vi "Write Sensor Servo Offset.vi"(7 "save to file (F)":bool, 8 "error in (no error)":errorcluster, 10 "ccw offset angle (rad)":dbl, 11 "starter kit host in":refnum<class "NI_Robotics_Starter Kit Host.lvclass">) -> (0 "error out":errorcluster, 3 "starter kit host out":refnum<class "NI_Robotics_Starter Kit Host.lvclass">)   [LabVIEW 2017, in "NI_Robotics_Starter Kit Host.lvclass"]
doc: "<B>Owning Palette:</B> Starter Kit 1.0 VIs, Starter Kit 2.0 VIs\n\nDefines the amount by which the zero, or straight-forward, position of the distance sensor differs from the zero position of the sensor servo on which the sensor is mounted. You can use this VI to save the offset value to a file so the value is associated with the same robot in the future."
uses:
  <vilib>/robotics/Starter Kit/Host Interface/NI_Robotics_Starter Kit Host.lvclass
  <vilib>/robotics/Starter Kit/Host Interface/NI_Robotics_Starter Kit Host.lvclass/NI_Robotics_Starter Kit Host.ctl
  <vilib>/robotics/Starter Kit/Servo Motor/NI_Robotics_Starter Kit Servo Motor.lvclass
  <vilib>/robotics/Utilities/NI_Robotics Utilities.lvlib
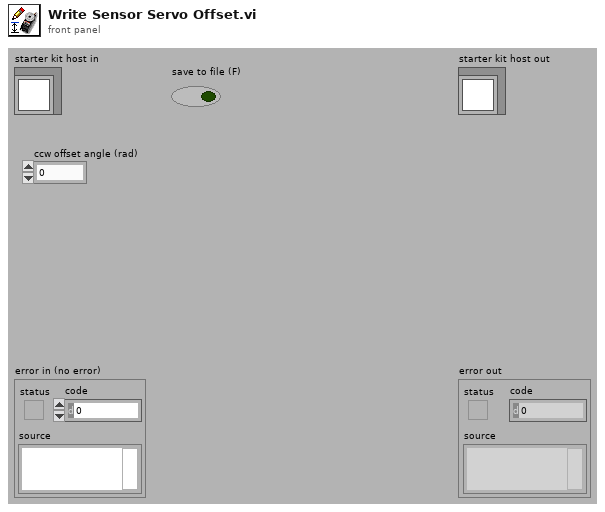
[diagram p1: front panel]
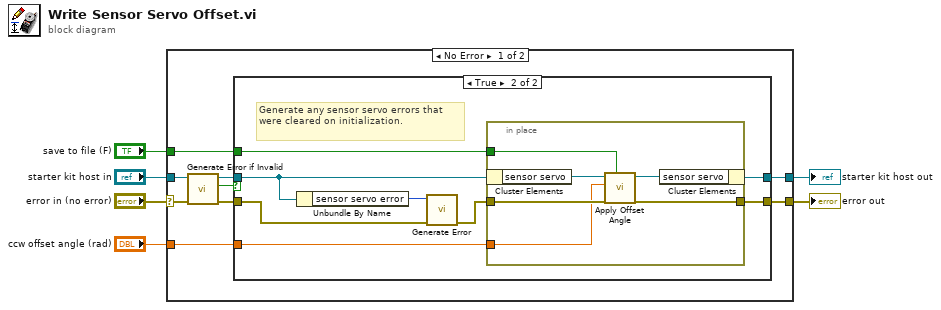
[diagram p0: block diagram]
diagram:
  n1 = case shown="No Error" "error in (no error)" {
    selector: "error in (no error)" -> [w9 w33]
    tunnel: [w14 w33] -> w5
    tunnel: [w15 w32] -> w3
    tunnel: "starter kit host in" -> [w11 w32]
    tunnel: "ccw offset angle (rad)" -> [w13 _]
    tunnel: "save to file (F)" -> [w12 _]
    frame No Error {
      n2 = call <vilib>:"Generate Error if Invalid.vi"("error in (no error)"=w9, "starter kit host in"=w11) -> ("error out"=w8:errorcluster, "valid?"=w7:bool, "starter kit host out"=w10:refnum<class "NI_Robotics_Starter Kit Host.lvclass">)  [unwired: 7 in]
      n3 = case shown="True" w7 {
        tunnel: [w17 w25] -> w15
        tunnel: [w16 w24] -> w14
        tunnel: w13 -> [_ w23]
        tunnel: w12 -> [_ w22]
        tunnel: w10 -> [w17 w18]
        tunnel: w8 -> [w16 w19]
        frame False {
        }
        frame True {
          # "Generate any sensor servo errors that were cleared on initialization."
          n4 = Unbundle By Name(w18) -> ("sensor servo error"=w21:i32)
          n5 = call <vilib>:"Generate Error.vi"("error in (no error)"=w19, "code"=w21) -> ("error out"=w20:errorcluster)  [unwired: 9 in]
          n6 = in-place {
            in-place-border: w20 -> [w29]
            in-place-border: [w28] -> w24
            in-place-border: w23 -> [w27]
            in-place-border: w22 -> [w26]
            n7 = in-place-cluster #1(w18) -> ("sensor servo"=w31:refnum<class "NI_Robotics_Starter Kit Servo Motor.lvclass">)
            n8 = call <vilib>:"Apply Offset Angle.vi"("save to file (F)"=w26, "error in (no error)"=w29, "ccw offset angle (rad)"=w27, "servo motor in"=w31) -> ("error out"=w28:errorcluster, "servo motor out"=w30:refnum<class "NI_Robotics_Starter Kit Servo Motor.lvclass">)  [unwired: 6 in]
            n9 = in-place-cluster #1("sensor servo"=w30) -> (w25:refnum<class "NI_Robotics_Starter Kit Host.lvclass">)
          }
        }
      }
    }
    frame Error {
    }
  }
  "error out" <- w5
  "starter kit host out" <- w3
